vi "Check_Position_PN.vi"(4 "Extrusion mode":bool, 5 "Collision mode":T1=enum."Traverse - All", 6 "Model Rotation (deg)":sgl[](array[numeric])=[0.0, 0.0, 0.0] format="%.2g", 7 "Traverse extruded position":sgl[](array[numeric])=[0.0, 0.0, 0.0] format="%.2g", 8 "Position to check":sgl[](array[numeric])=[0.0, 0.0, 0.0] format="%.2g", 9 "Traverse Name":string) -> (1 "Collision":bool, 3 "Error Comments":string)   [LabVIEW 2014]
uses:
  Collision_Detection/Triangles/EnFlo specific/Collision Mode.ctl
  <vilib>/Analysis/baseanly.llb/Unit Vector (DBL).vi
  <vilib>/Analysis/_algsub.llb/Real Vector Norm.vi
  Globals/Constants_global.vi
  <vilib>/Analysis/NI_AALBase.lvlib
  <vilib>/Analysis/NI_AALPro.lvlib
panel:
  # "X\n\nY\n\nZ"
  # "Roll\n\nPitch\n\nYaw"
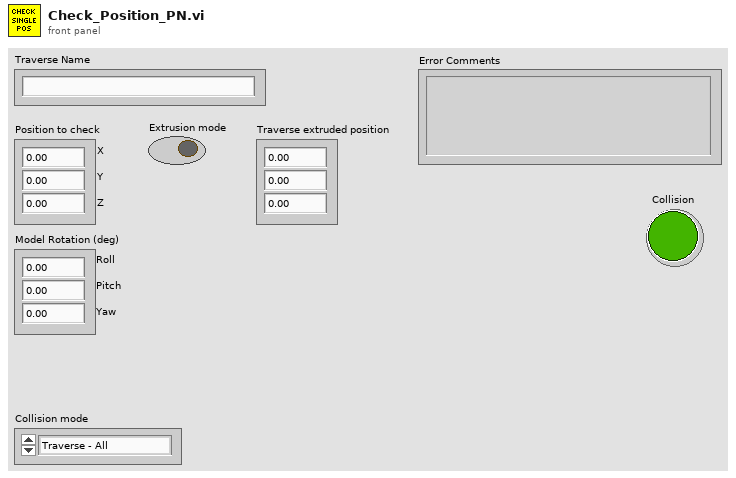
[diagram p1: front panel]
types:
  T1 = typedef "Collision Mode.ctl" = enum16{"Traverse - Tunnel", "Traverse - Model", "Traverse - Traverse", "Traverse - All"}
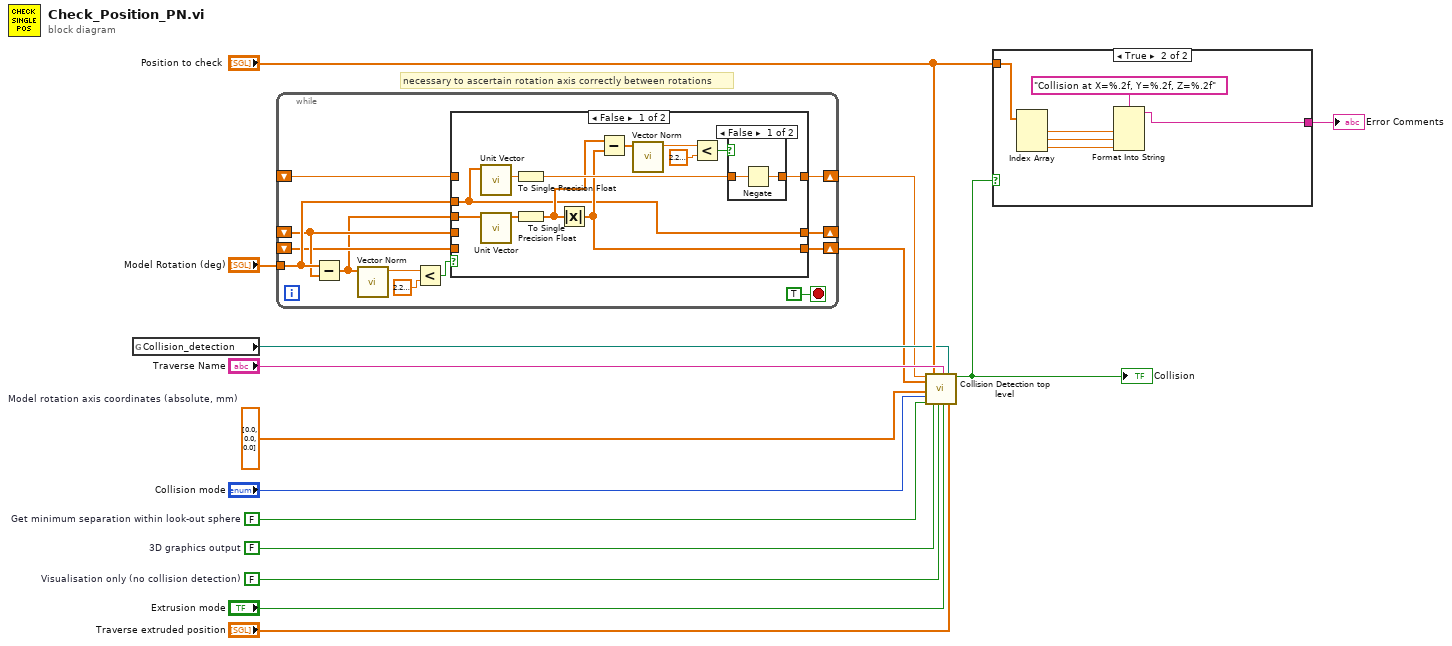
[diagram p0: block diagram]
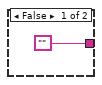
[diagram p4: hidden frame]
diagram:
  w1 = FALSE  # Get minimum separation within look-out sphere
  w6 = FALSE  # 3D graphics output
  w4 = FALSE  # Visualisation only (no collision detection)
  w15 = sgl[] [0.0, 0.0, 0.0]  # Model rotation axis coordinates (absolute, mm)
  # "necessary to ascertain rotation axis correctly between rotations"
  n1 = global read "Constants_global.vi" "Collision_detection"() -> (w10:path)
  n2 = while {
    shift-right: [w22] -> _
    shift-left: _ -> [w23]
    tunnel: "Model Rotation (deg)" -> [w24]
    shift-right: [w26] -> w8
    shift-left: _ -> [w21]
    shift-right: [w20] -> w7
    shift-left: _ -> [w19]
    stop <- TRUE stop-if-true
    n3 = Subtract(x=w24, y=w23) -> (x-y=w17:sgl[])
    n4 = call-poly <vilib>:"Vector Norm.vi"("Input Vector"=w17) -> ("norm"=w16:dbl)  [unwired: 9 in, 1 out]
    n5 = Less?(x=w16, y=2.220446049250313e-16) -> (x < y?=w18:bool)
    n6 = case shown="False" w18 {
      tunnel: w24 -> [w30 _]
      tunnel: w23 -> [_ w45]
      tunnel: [w32 w44] -> w26
      tunnel: [w30 w45] -> w22
      tunnel: w21 -> [_ w44]
      tunnel: w17 -> [w38 _]
      tunnel: [w31 w43] -> w20
      tunnel: w19 -> [_ w43]
      frame False {
        n7 = call-poly <vilib>:"Unit Vector.vi"("Input Vector"=w30) -> ("norm"=w34:dbl)  [unwired: 8 in, 2 out]
        n8 = call-poly <vilib>:"Unit Vector.vi"("Input Vector"=w38) -> ("Unit Vector"=w39:dbl[])  [unwired: 8 in, 2 out]
        n9 = To Single Precision Float(number=w34) -> (single precision float=w35:sgl)
        n10 = To Single Precision Float(number=w39) -> (single precision float=w33:sgl[])
        n11 = Absolute Value(x=w33) -> (abs(x)=w32:sgl[])
        n12 = Subtract(x=w33, y=w32) -> (x-y=w29:sgl[])
        n13 = call-poly <vilib>:"Vector Norm.vi"("Input Vector"=w29) -> ("norm"=w28:dbl)  [unwired: 9 in, 1 out]
        n14 = Less?(x=w28, y=2.220446049250313e-16) -> (x < y?=w36:bool)
        n15 = case shown="False" w36 {
          tunnel: [w40 w42] -> w31
          tunnel: w35 -> [w41 w42]
          frame False {
            n16 = Negate(x=w41) -> (-x=w40:sgl)
          }
          frame True {
          }
        }
      }
      frame True {
      }
    }
  }
  n17 = call "Collision Detection top level.vi"("Model rotation (absolute, degrees)"=w7, "Model rotation axis (unit vector)"=w8, "Model rotation axis coordinates (absolute, mm)"=w15, "Collision mode"="Collision mode", "Get minimum separation within look-out sphere"=w1, "Traverse position (absolute, mm)"="Position to check", "3D graphics output"=w6, "Visualisation only (no collision detection)"=w4, "Traverse name"="Traverse Name", "Extrusion mode"="Extrusion mode", "Rig geometry directory path"=w10, "Traverse extruded position"="Traverse extruded position") -> ("Collision"=w13:bool)  [unwired: 3 in, 4 out]
  "Collision" <- w13
  n18 = case shown="True" w13 {
    tunnel: "Position to check" -> [_ w52]
    tunnel: ["" w47] -> w11
    frame False {
    }
    frame True {
      n19 = Index Array(array=w52) -> (element #1=w51:sgl, element #2=w50:sgl, element #3=w49:sgl)  [unwired: 3 in]
      n20 = Format Into String(format string="Collision at X=%.2f, Y=%.2f, Z=%.2f", w51, w50, w49) -> (resulting string=w47:string)  [unwired: 2 in, 1 out]
    }
  }
  "Error Comments" <- w11
